vi "initialise.vi"(8 "error in (no error)":errorcluster, 11 "NetworkPixelfly in":refnum<class "NetworkPixelfly.lvclass">) -> (0 "error out":errorcluster, 3 "NetworkPixelfly out":refnum<class "NetworkPixelfly.lvclass">)   [LabVIEW 2009, in "Hardware.lvlib" / "HWControllers.lvlib" / "NetworkPixelfly.lvclass"]
uses:
  NetworkPixelfly.lvclass
  Channels/Camera/PixelflySA/PixelflySA.lvclass
  NetworkPixelfly.lvclass/NetworkPixelfly.ctl
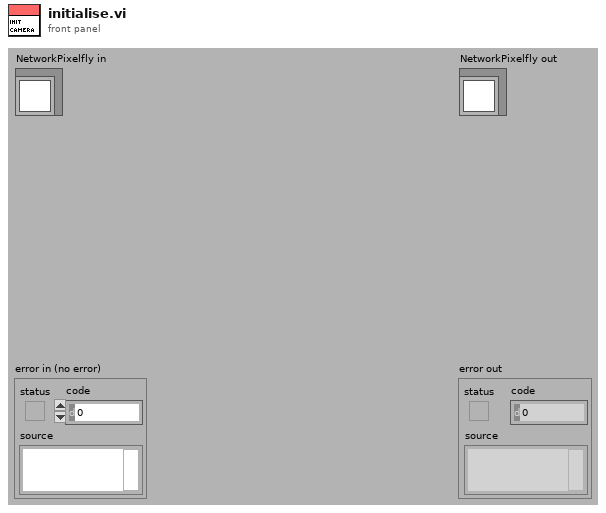
[diagram p1: front panel]
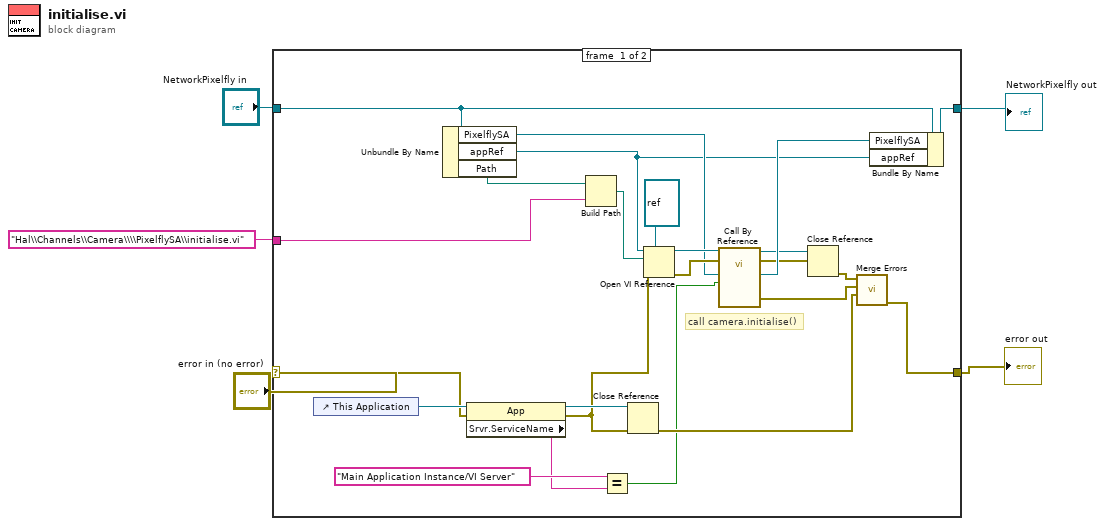
[diagram p0: block diagram]
diagram:
  n1 = case shown="No Error" "error in (no error)" {
    selector: "error in (no error)" -> [w9 w31]
    tunnel: [w15 w31] -> w2
    tunnel: [w14 w30] -> w1
    tunnel: "NetworkPixelfly in" -> [w22 w30]
    tunnel: "Hal\\Channels\\Camera\\\\PixelflySA\\initialise.vi" ("viPath") -> [w28 _]
    frame #0 {
      # "call camera.initialise()"
      n2 = control-ref of="This Application"() -> (w13:refnum<vi>)
      n3 = Unbundle By Name(w22) -> ("PixelflySA"=w23:refnum<class "PixelflySA.lvclass">, "appRef"=w20:refnum<vi>, "Path"=w27:path)
      n4 = property class="App"(reference=w13, error in=w9) -> (reference out=w12:refnum<vi>, error out=w8:errorcluster, "Srvr.ServiceName"=w10:string)
      n5 = Build Path(base path=w27, name or relative path=w28) -> (appended path=w29:path)
      n6 = Equal?(x="Main Application Instance/VI Server", y=w10) -> (x = y?=w6:bool)
      n7 = Close Reference(reference=w12, error in (no error)=w8) -> (error out=w7:errorcluster)
      n8 = Open VI Reference(type specifier VI Refnum (for type only)=refnum<vi> refnum, application reference (local)=w20, vi path=w29, error in (no error)=w8) -> (vi reference=w25:refnum<vi>, error out=w24:errorcluster)  [unwired: 2 in]
      n9 = call-by-ref "?"(reference=w25, error in=w24, "main_app_instance"=w6, "Pixelfly in"=w23) -> (reference out=w19:refnum<vi>, error out=w18:errorcluster, 0:"error out"=w16:errorcluster, "Pixelfly out"=w21:refnum<class "PixelflySA.lvclass">)  [unwired: 8 in]
      n10 = Close Reference(reference=w19, error in (no error)=w18) -> (error out=w17:errorcluster)
      n11 = call <vilib>:"Merge Errors.vi"("error in 3 (no error)"=w7, "error in 2 (no error)"=w16, "error in 1 (no error)"=w17) -> ("error out"=w15:errorcluster)  [unwired: 4 in]
      n12 = Bundle By Name(cluster=w22, "PixelflySA"=w21, "appRef"=w20) -> (w14:refnum<class "NetworkPixelfly.lvclass">)
    }
    frame #1 {
    }
  }
  "error out" <- w2
  "NetworkPixelfly out" <- w1
